vi "BackgroundSubstraction.vi"(10 "Background Refnum":refnum<vi>, 11 "ROI Refnum":refnum<vi>) -> (3 "Background Sub ROI":dbl[][](graph))   [LabVIEW 2014]
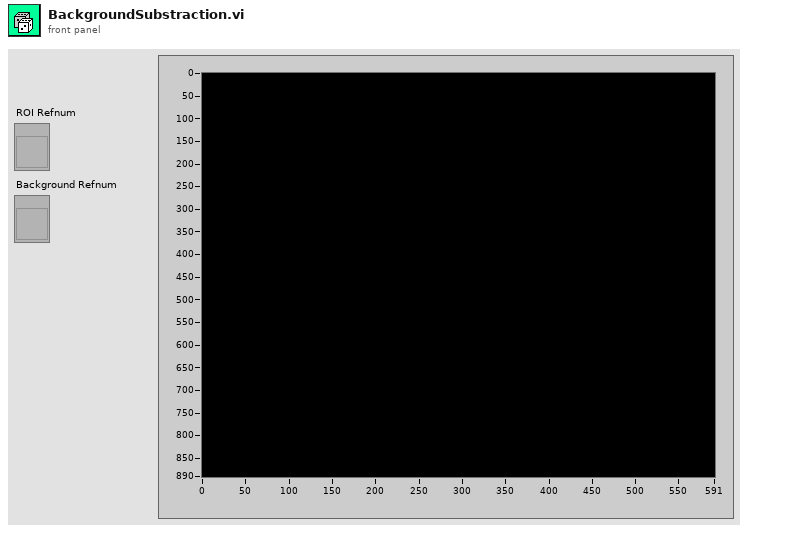
[diagram p1: front panel]
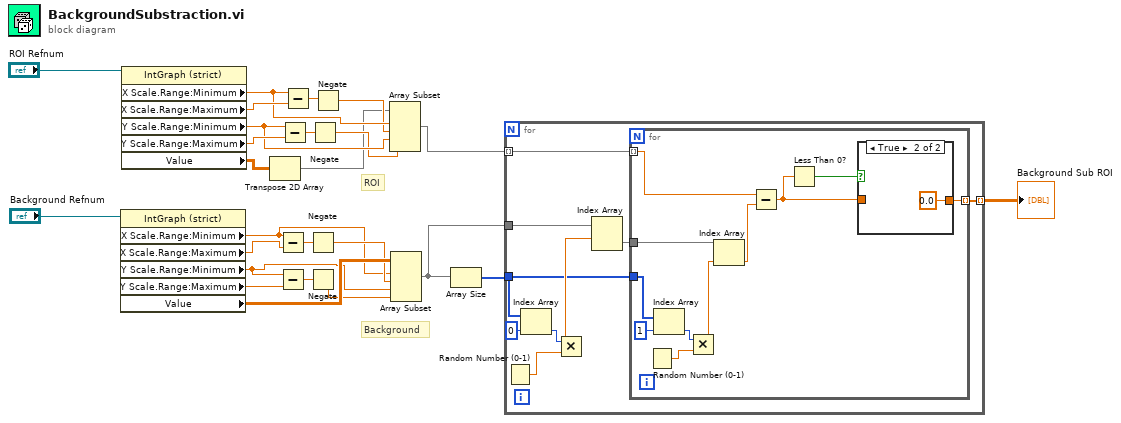
[diagram p0: block diagram]
diagram:
  # "ROI"
  # "Background"
  n1 = property on="Property Node" class="IntGraph (strict)"(reference="Background Refnum") -> ("X Scale.Range:Minimum"=w9:dbl, "X Scale.Range:Maximum"=w17:dbl, "Y Scale.Range:Minimum"=w8:dbl, "Y Scale.Range:Maximum"=w16:dbl, "Value"=w11:dbl[][])  [unwired: 1 in, 2 out]
  n2 = property on="Property Node" class="IntGraph (strict)"(reference="ROI Refnum") -> ("X Scale.Range:Minimum"=w15:dbl, "X Scale.Range:Maximum"=w23:dbl, "Y Scale.Range:Minimum"=w13:dbl, "Y Scale.Range:Maximum"=w22:dbl, "Value"=w4:dbl[][])  [unwired: 1 in, 2 out]
  n3 = Transpose 2D Array(2D array=w4) -> (transposed array=w3:dbl[][])
  n4 = Subtract(x=w9, y=w17) -> (x-y=w19:dbl)
  n5 = Subtract(x=w8, y=w16) -> (x-y=w18:dbl)
  n6 = Subtract(x=w13, y=w22) -> (x-y=w20:dbl)
  n7 = Subtract(x=w15, y=w23) -> (x-y=w21:dbl)
  n8 = Negate(x=w19) -> (-x=w10:dbl)
  n9 = Negate(x=w18) -> (-x=w7:dbl)
  n10 = Negate(x=w20) -> (-x=w12:dbl)
  n11 = Negate(x=w21) -> (-x=w14:dbl)
  n12 = Array Subset(array=w3, index (row)=w15, length (row)=w14, index (col)=w13, length (col)=w12) -> (w2:dbl[][])
  n13 = Array Subset(array=w11, index (row)=w9, length (row)=w10, index (col)=w8, length (col)=w7) -> (w6:dbl[][])
  n14 = Array Size(array=w6) -> (size(s)=w5:i32[])
  n15 = for {
    tunnel: w2 -> [w34] mode=indexing
    tunnel: w6 -> [w33]
    tunnel: w5 -> [w27]
    tunnel: [w26] -> w1 mode=indexing
    n16 = Random Number (0-1)() -> (number: 0 to 1=w32:dbl)
    n17 = Index Array(array=w27, index=0) -> (element=w30:i32)
    n18 = Multiply(x=w30, y=w32) -> (x*y=w29:dbl)
    n19 = Index Array(array=w33, index (row)=w29) -> (element=w28:dbl[])  [unwired: 1 in]
    n20 = for {
      tunnel: w34 -> [w39] mode=indexing
      tunnel: w28 -> [w41]
      tunnel: w27 -> [w42]
      tunnel: [w35] -> w26 mode=indexing
      n21 = Random Number (0-1)() -> (number: 0 to 1=w45:dbl)
      n22 = Index Array(array=w42, index=1) -> (element=w43:i32)
      n23 = Multiply(x=w43, y=w45) -> (x*y=w40:dbl)
      n24 = Index Array(array=w41, index=w40) -> (element=w38:dbl)
      n25 = Subtract(x=w39, y=w38) -> (x-y=w36:dbl)
      n26 = Less Than 0?(x=w36) -> (x < 0?=w37:bool)
      n27 = case shown="True" w37 {
        tunnel: w36 -> [w46 _]
        tunnel: [w46 0.0] -> w35
        frame False {
        }
        frame True {
        }
      }
    }
  }
  "Background Sub ROI" <- w1
